vi "MD5.vi"(10 "data":u8[](array[numeric]) format="%02x") -> (2 "MD5 hash":u8[](array[numeric]) format="%02x")   [LabVIEW 2013, in "MD5.lvlib"]
uses:
  MD5.lvlib
  MD5.lvclass
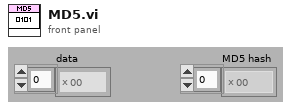
[diagram p1: front panel]
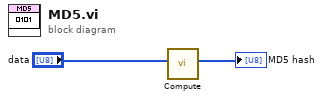
[diagram p0: block diagram]
diagram:
  n1 = call "Compute.vi"("data"="data") -> ("hash"=→"MD5 hash":u8[])  [unwired: 10 in]
